vi "Obtain Writer.vi"(10 "Qt Type":string, 11 "Class Ref Map":T1) -> (1 "Type Supported?":bool, 2 "Param Writer":refnum<class "Abstract Param Writer.lvclass">)   [LabVIEW 2013]
uses:
  Abstract Param Writer/Abstract Param Writer.lvclass
  <userlib>/ICON Technologies/ICON Maps/lvlib/Map.ctl
  Bool Writer/Bool Writer.lvclass
  String Writer/String Writer.lvclass
  QObject Writer/QObject Writer.lvclass
  QObject Writer/QObject Writer.lvclass/QObject Writer.ctl
  <userlib>/ICON Technologies/ICON Maps/ICON Maps.lvlib
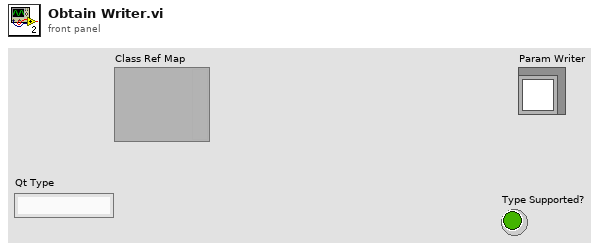
[diagram p1: front panel]
types:
  T1 = typedef "ICON Maps.lvlib/Map.ctl" = variant
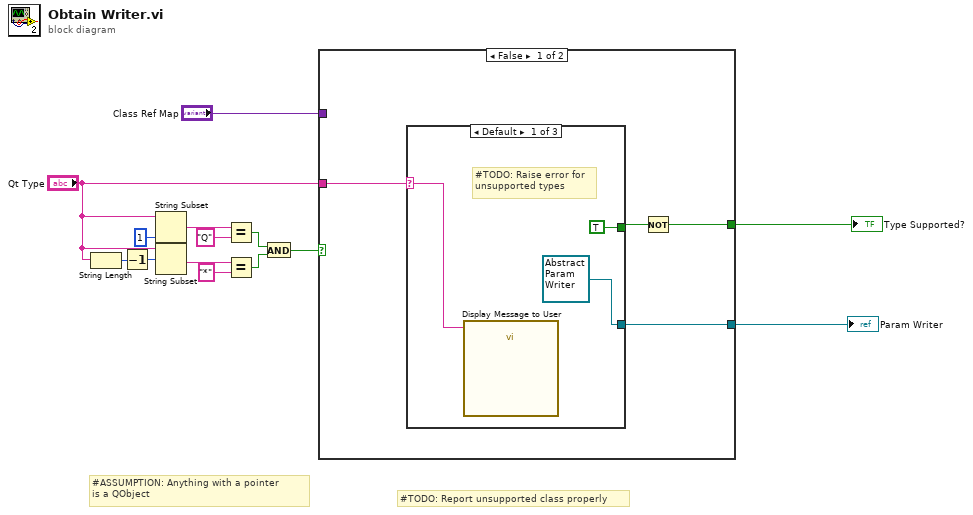
[diagram p0: block diagram]
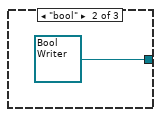
[diagram p2: hidden frame]
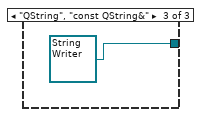
[diagram p3: hidden frame]
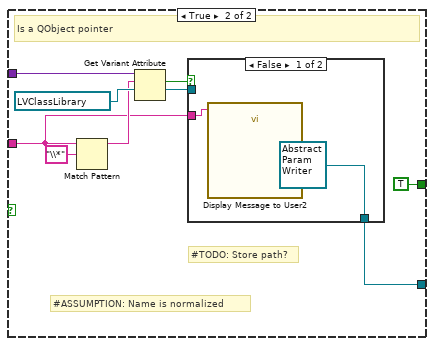
[diagram p4: hidden frame]
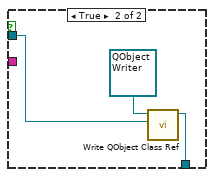
[diagram p5: hidden frame]
diagram:
  # "#TODO: Report unsupported class properly"
  # "#ASSUMPTION: Anything with a pointer\nis a QObject"
  n1 = String Length(string="Qt Type") -> (length=w12:i32)
  n2 = Decrement(x=w12) -> (x-1=w11:i32)
  n3 = String Subset(string="Qt Type", length (rest)=1 ("offset (0)")) -> (substring=w10:string)  [unwired: 1 in]
  n4 = String Subset(string="Qt Type", offset (0)=w11) -> (substring=w9:string)  [unwired: 1 in]
  n5 = Equal?(x=w10, y="Q") -> (x = y?=w6:bool)
  n6 = Equal?(x=w9, y="*") -> (x = y?=w5:bool)
  n7 = And(x=w6, y=w5) -> (x .and. y?=w4:bool)
  n8 = case shown="False" w4 {
    tunnel: [w17 TRUE] -> w14
    tunnel: "Qt Type" -> [w16 w24]
    tunnel: [w15 w31] -> w3
    tunnel: "Class Ref Map" -> [_ w29]
    frame False {
      n9 = case shown="Default" w16 {
        selector: w16 -> [w21 _ _]
        tunnel: [refnum<class "Abstract Param Writer.lvclass"> refnum ("Abstract Param Writer.lvclass") refnum<class "Bool Writer.lvclass"> refnum ("Bool Writer.lvclass") refnum<class "String Writer.lvclass"> refnum ("String Writer.lvclass")] -> w15
        tunnel: [TRUE _ _] -> w18
        frame Default {
          # "#TODO: Raise error for\nunsupported types"
          n10 = call "Display Message to User"("Message"=w21) -> ()  [unwired: 9 in, 2 out]
        }
        frame "bool" {
        }
        frame "QString", "const QString&" {
        }
      }
      n11 = Not(x=w18) -> (.not. x?=w17:bool)
    }
    frame True {
      # "#TODO: Store path?"
      # "#ASSUMPTION: Name is normalized"
      # "Is a QObject pointer"
      n12 = Match Pattern(string=w24, regular expression="\\*") -> (before substring=w27:string)  [unwired: 1 in, 3 out]
      n13 = Get Variant Attribute(Variant=w29, name=w27, default value (empty Variant)=refnum<vi> refnum ("specific class reference")) -> (found=w25:bool, value=w26:refnum<vi>)  [unwired: 1 in, 2 out]
      n14 = case shown="False" w25 {
        tunnel: [refnum<class "Abstract Param Writer.lvclass"> refnum ("Abstract Param Writer.lvclass") w36] -> w31
        tunnel: w26 -> [_ w35]
        tunnel: w24 -> [w33 _]
        frame False {
          n15 = call "Display Message to User2"("Message"=w33) -> ()  [unwired: 9 in, 2 out]
        }
        frame True {
          n16 = call "Write QObject Class Ref.vi"("QObject Class Ref"=w35, "QObject Writer in"=refnum<class "QObject Writer.lvclass"> refnum ("QObject Writer.lvclass")) -> ("QObject Writer out"=w36:refnum<class "QObject Writer.lvclass">)  [unwired: 8 in, 1 out]
        }
      }
    }
  }
  "Param Writer" <- w3
  "Type Supported?" <- w14
